vi "Start functions.vi"(8 "error in (no error)":errorcluster, 11 "Programming Logic in":refnum<class "Programming Logic.lvclass">) -> (0 "error out":errorcluster, 3 "Programming Logic out":refnum<class "Programming Logic.lvclass">)   [LabVIEW 2014, in "Files Library.lvlib" / "Programming Logic.lvclass"]
uses:
  Programming Logic.lvclass
  <vilib>/NI/Modbus Library/API/Master/Modbus Master.lvclass
panel:
  in  "Time Limit":u16
  in  "Temperature Setpoint":u16
  in  "Speed":u16
  in  "Start":bool
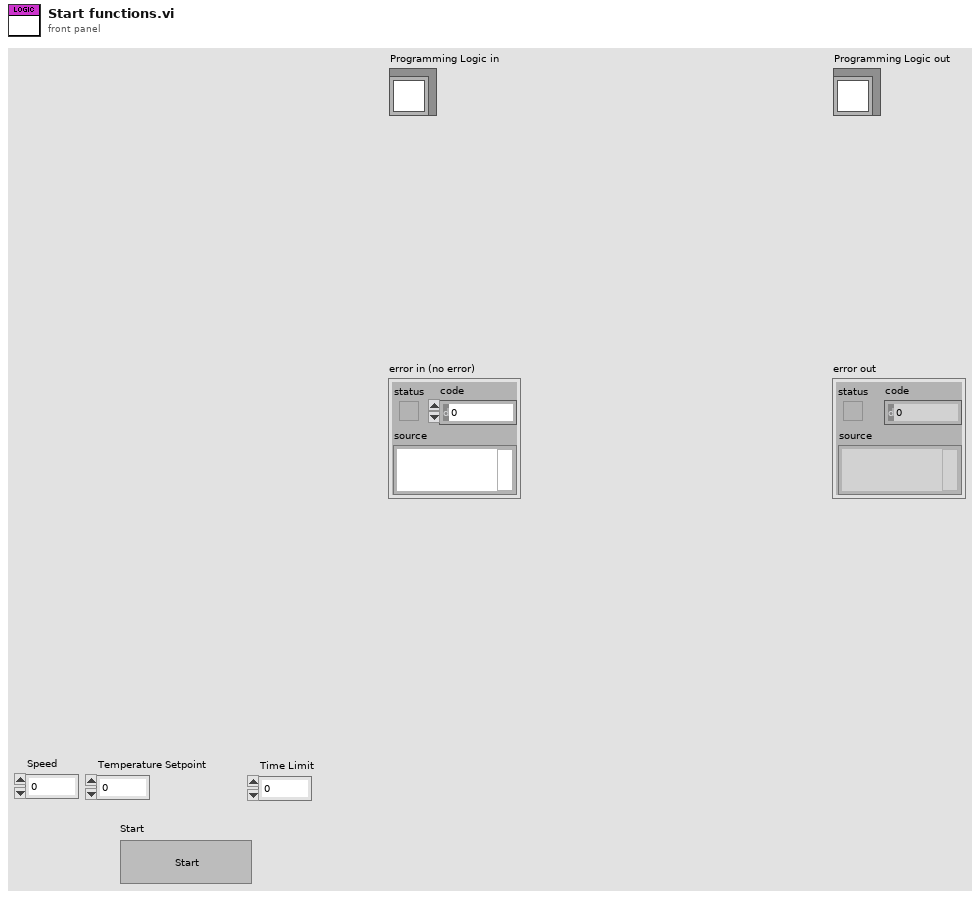
[diagram p1: front panel]
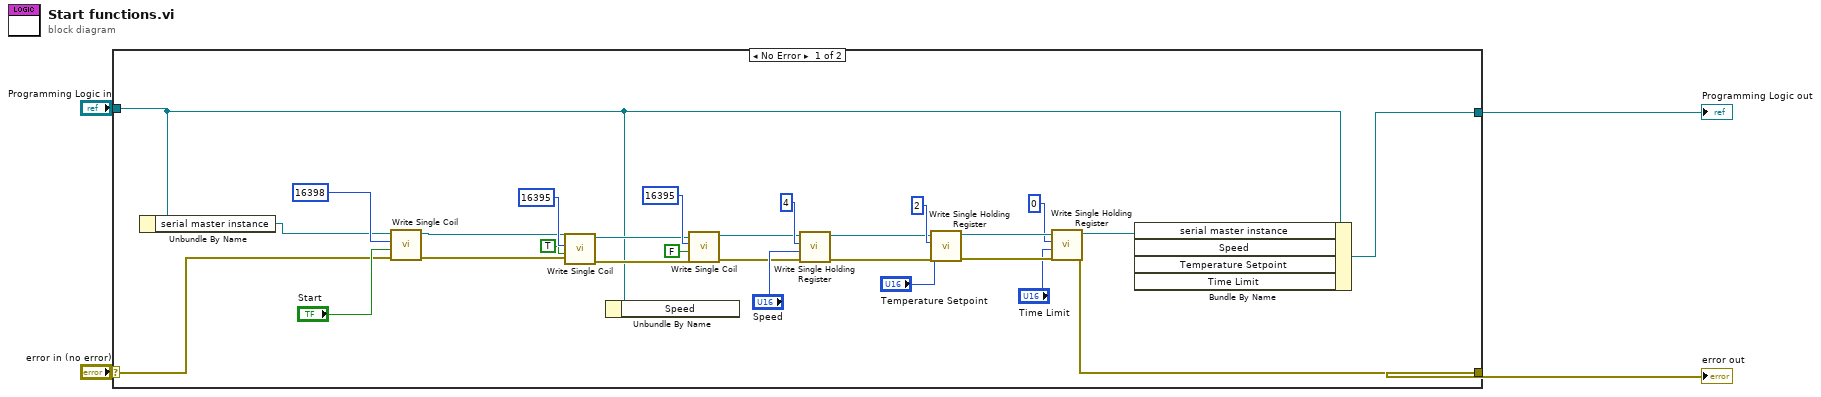
[diagram p0: block diagram]
diagram:
  n1 = case shown="No Error" "error in (no error)" {
    selector: "error in (no error)" -> [w10 w34]
    tunnel: [w9 w34] -> w3
    tunnel: [w6 w33] -> w1
    tunnel: "Programming Logic in" -> [w5 w33]
    frame No Error {
      n2 = Unbundle By Name(w5) -> ("serial master instance"=w8:refnum<class "Modbus Master.lvclass">)
      n3 = call-dynamic "Write Single Coil.vi"("error in"=w10, "coil to write"="Start", "address"=u16 16398, "Modbus master in"=w8) -> ("error out"=w24:errorcluster, "Modbus master out"=w26:refnum<class "Modbus Master.lvclass">)  [unwired: 6 in]
      n4 = call-dynamic "Write Single Coil.vi"("error in"=w24, "coil to write"=TRUE, "address"=u16 16395, "Modbus master in"=w26) -> ("error out"=w23:errorcluster, "Modbus master out"=w25:refnum<class "Modbus Master.lvclass">)  [unwired: 6 in]
      n5 = Unbundle By Name(w5) -> ()  [unwired: 1 out]
      n6 = call-dynamic "Write Single Coil.vi"("error in"=w23, "coil to write"=FALSE, "address"=u16 16395, "Modbus master in"=w25) -> ("error out"=w17:errorcluster, "Modbus master out"=w18:refnum<class "Modbus Master.lvclass">)  [unwired: 6 in]
      n7 = call-dynamic "Write Single Holding Register.vi"("error in"=w17, "register to write"="Speed", "address"=u16 4, "Modbus master in"=w18) -> ("error out"=w15:errorcluster, "Modbus master out"=w16:refnum<class "Modbus Master.lvclass">)  [unwired: 6 in]
      n8 = call-dynamic "Write Single Holding Register.vi"("error in"=w15, "register to write"="Temperature Setpoint", "address"=u16 2, "Modbus master in"=w16) -> ("error out"=w13:errorcluster, "Modbus master out"=w14:refnum<class "Modbus Master.lvclass">)  [unwired: 6 in]
      n9 = call-dynamic "Write Single Holding Register.vi"("error in"=w13, "register to write"="Time Limit", "address"=u16 0, "Modbus master in"=w14) -> ("error out"=w9:errorcluster, "Modbus master out"=w7:refnum<class "Modbus Master.lvclass">)  [unwired: 6 in]
      n10 = Bundle By Name(cluster=w5, "serial master instance"=w7) -> (w6:refnum<class "Programming Logic.lvclass">)  [unwired: 3 in]
    }
    frame Error {
    }
  }
  "error out" <- w3
  "Programming Logic out" <- w1
